vi "SetWavelength.vi"(8 "error in":errorcluster, 9 "wavelength":dbl, 10 "Slit":string, 11 "Port":refnum<visa-resource-name>) -> (0 "error out":errorcluster, 3 "Port out":refnum<visa-resource-name>)   [LabVIEW 2018]
uses:
  Strict Type Controls/Settings Operation.ctl
  classes/Variable Manager/VariableManager_Bool.vi
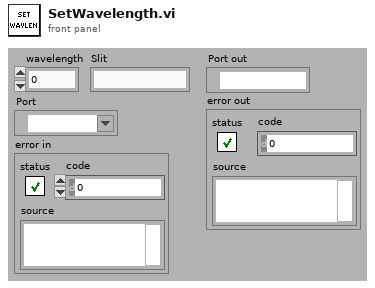
[diagram p1: front panel]
types:
  T1 = typedef "Settings Operation.ctl" = enum8{"Get Value", "Set Value", "Read File", "Write File", "Write Stored Value"}
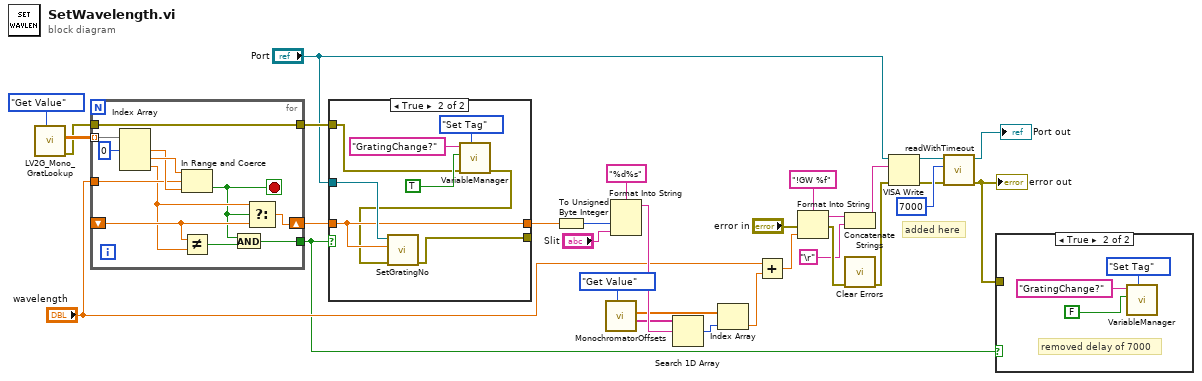
[diagram p0: block diagram]
diagram:
  # "added here"
  n1 = call "LV2G_Mono_GratLookup.vi"("Operation"=Settings_Operation."Get Value") -> ("error out"=w12:errorcluster, "lookupOut1"=w19:dbl[][])  [unwired: 8 in, 1 out]
  n2 = for {
    tunnel: w19 -> [w43] mode=indexing
    tunnel: "wavelength" -> [w39]
    shift-right: [w34] -> w16
    shift-left: _ -> [w38]
    tunnel: [w33] -> w14
    tunnel: w12 -> [w32]
    tunnel: [w32] -> w11
    stop <- w35 stop-if-true
    n3 = Index Array(array=w43, index #1=0 ("index")) -> (element #1=w40:dbl, element #2=w41:dbl, element #3=w37:dbl)  [unwired: 2 in]
    n4 = In Range and Coerce(upper limit=w41, x=w39, lower limit=w40) -> (In Range?=w35:bool)  [unwired: 1 out]
    n5 = Not Equal?(x=w38, y=w37) -> (x != y?=w36:bool)
    n6 = And(x=w35, y=w36) -> (x .and. y?=w33:bool)
    n7 = Select(t=w37, s=w35, f=w38) -> (s? t:f=w34:dbl)
  }
  n8 = case shown="True" w14 {
    tunnel: w16 -> [w45 w49]
    tunnel: [w45 w49] -> w15
    tunnel: "Port" -> [_ w50]
    tunnel: w11 -> [w44 w48]
    tunnel: [w44 w46] -> _
    frame False {
    }
    frame True {
      n9 = call-poly "VariableManager.vi"("Operation"=enum16{"Get Tag", "Set Tag"}."Set Tag", "error in (no error)"=w48, "Value"=TRUE, "Tag"="GratingChange?") -> ("error out"=w47:errorcluster)  [unwired: 4 in, 3 out]
      n10 = call "SetGratingNo.vi"("error in"=w47, "GratingNo"=w49, "Port"=w50) -> ("error out"=w46:errorcluster)  [unwired: 6 in, 2 out]
    }
  }
  n11 = To Unsigned Byte Integer(number=w15) -> (unsigned 8bit integer=w17:u8)
  n12 = call "MonochromatorOffsets.vi"("Operation"=Settings_Operation."Get Value") -> ("Channel"=w26:string[], "offsets"=w25:dbl[])  [unwired: 7 in, 2 out]
  n13 = Format Into String(format string="%d%s", w17, "Slit") -> (resulting string=w27:string)  [unwired: 2 in, 1 out]
  n14 = Search 1D Array(1D array=w26, element=w27) -> (index of element=w24:i32)  [unwired: 1 in]
  n15 = Index Array(array=w25, index=w24) -> (element=w21:dbl)
  n16 = Add(x="wavelength", y=w21) -> (x+y=w20:dbl)
  n17 = Format Into String(format string="!GW %f" ("concatenated string"), error in="error in", w20) -> (resulting string=w30:string, error out=w10:errorcluster)  [unwired: 1 in]
  n18 = Concatenate Strings(w30, "\r") -> (w8:string)
  n19 = call <vilib>:"Clear Errors.vi"("error in (no error)"=w10) -> ("error out"=w9:errorcluster)  [unwired: 5 in, 1 out]
  n20 = VISA Write(VISA resource name="Port", write buffer=w8, error in (no error)=w9) -> (VISA resource name out=w6:refnum<visa-resource-name>, error out=w3:errorcluster)  [unwired: 1 out]
  n21 = call "readWithTimeout.vi"("error in"=w3, "timeOut"=u32 7000, "Port"=w6) -> ("error out"=w2:errorcluster, "Port out"=→"Port out":refnum<visa-resource-name>)  [unwired: 6 in, 1 out]
  "error out" <- w2
  n22 = case shown="True" w14 {
    tunnel: w2 -> [_ _]
    frame False {
    }
    frame True {
      # "removed delay of 7000"
      n23 = call-poly "VariableManager.vi"("Operation"=enum16{"Get Tag", "Set Tag"}."Set Tag", "Value"=FALSE, "Tag"="GratingChange?") -> ()  [unwired: 5 in, 4 out]
    }
  }
